vi "fileObjectivesRegistrationLoad.vi"(0 "objectiveRegistrationFilePath":string) -> (4 "denormParam":dbl[](array[numeric]), 5 "z(opto)z(img)":dbl[][](array[numeric]), 6 "param":dbl[](array[numeric]), 7 "imaging (model)":dbl[][](array[numeric]), 8 "normParam":dbl[](array[numeric]), 9 "optogenetics (scene)":dbl[][](array[numeric]))   [LabVIEW 2017]
uses:
  <vilib>/Utility/file.llb/Read Delimited Spreadsheet (DBL).vi
  <vilib>/Analysis/polynomials.llb/1D Polynomial Evaluation (DBL).vi
  globalUtilities.vi
  <vilib>/Analysis/NI_AALPro.lvlib
panel:
  out "Array":dbl[][][](array[numeric])
  out "f":string
  out "XY Graph":T1(graph)
  out "dtp1(dpt0)":dbl[](array[numeric])
  out "dtp0(dpt1)":dbl[](array[numeric])
  # "a1"
  # "a0"
  # "a2"
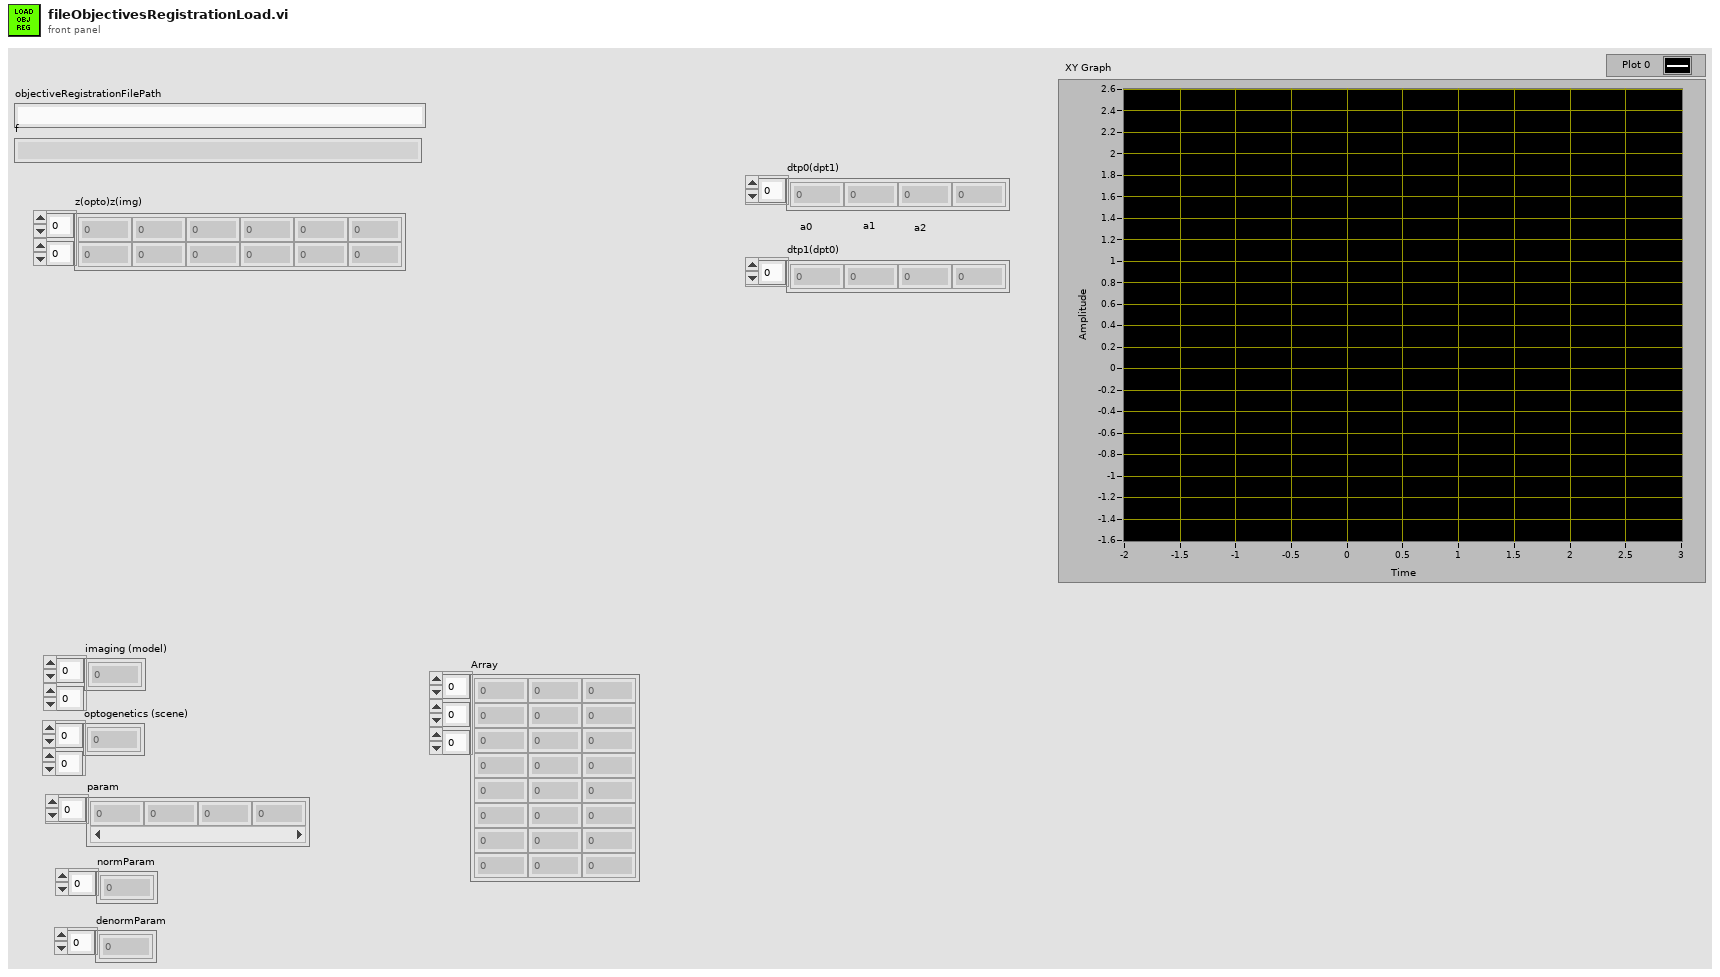
[diagram p1: front panel]
types:
  T1 = cluster{"all rows":dbl[], "Best Polynomial Fit":dbl[]}[]
  T2 = cluster{"all rows":dbl[], "Best Polynomial Fit":dbl[]}
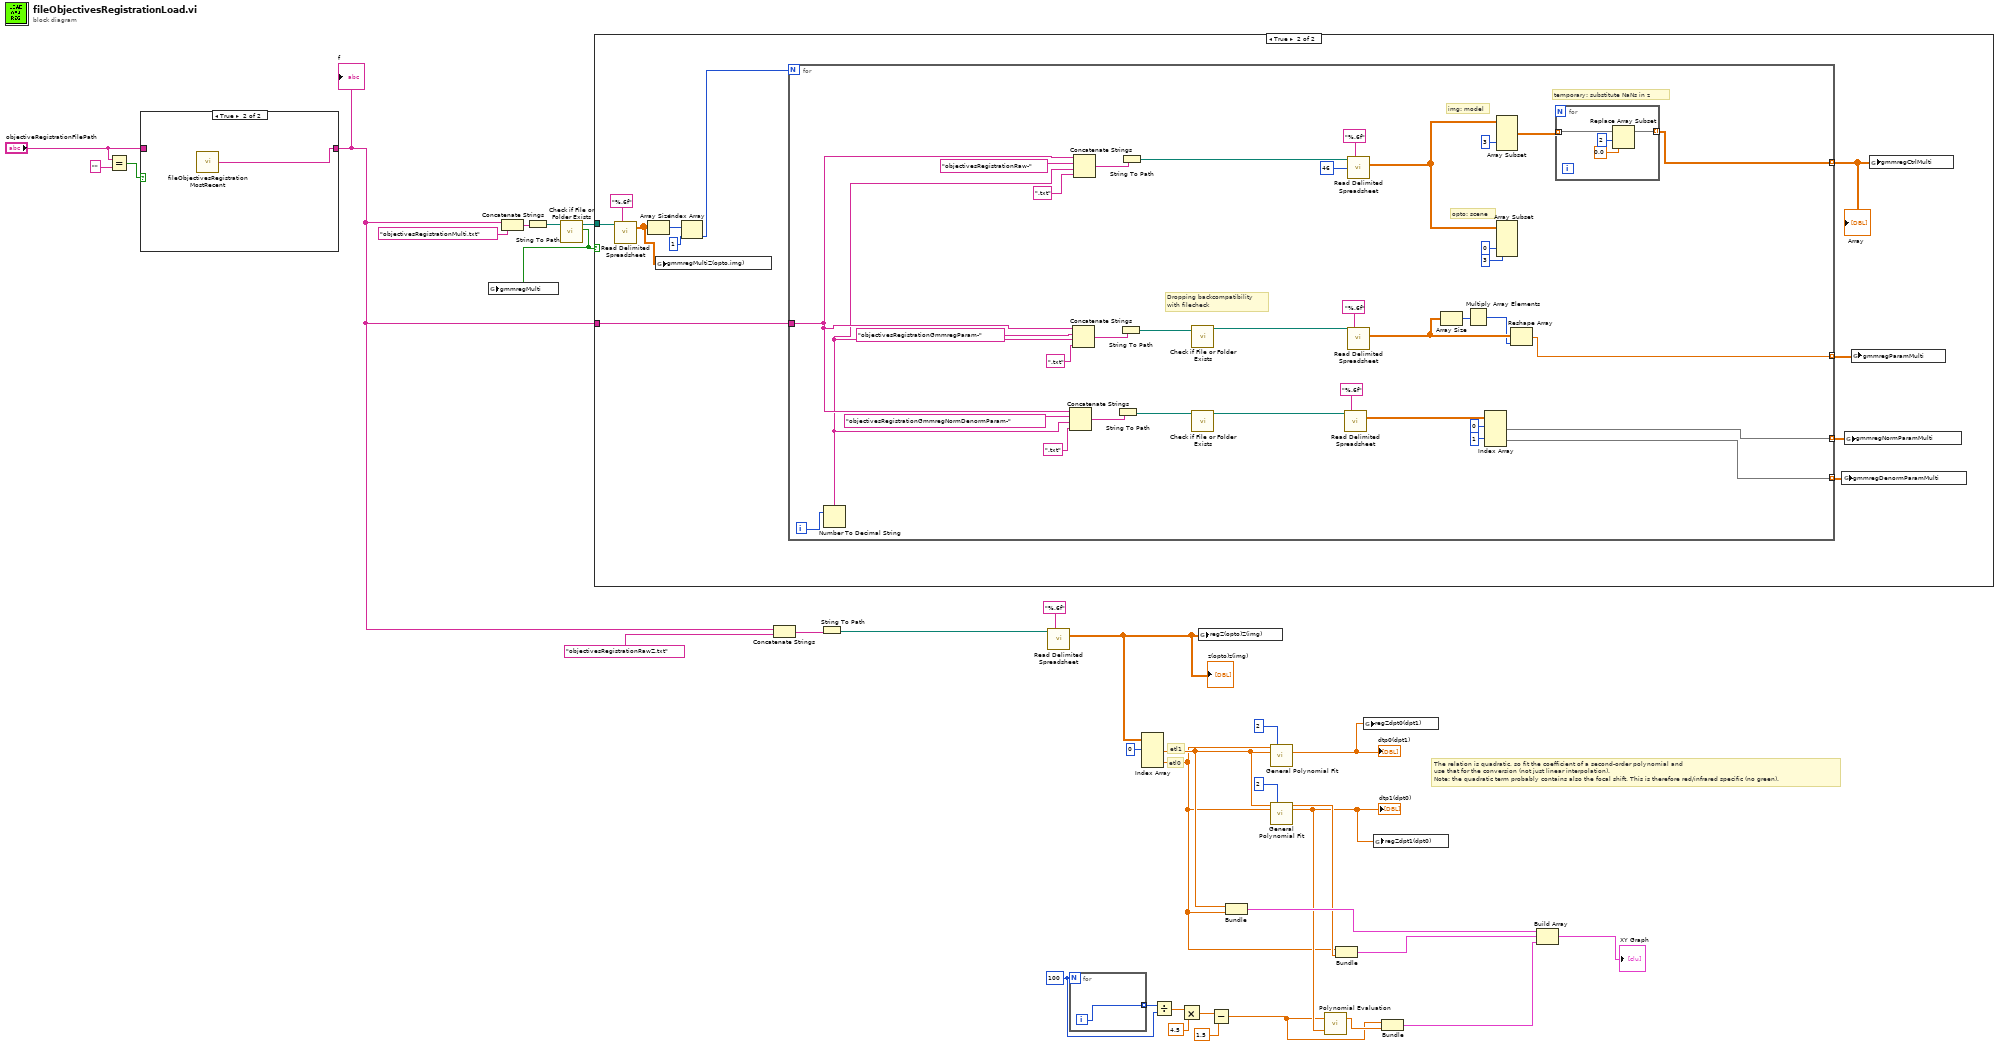
[diagram p0: block diagram]
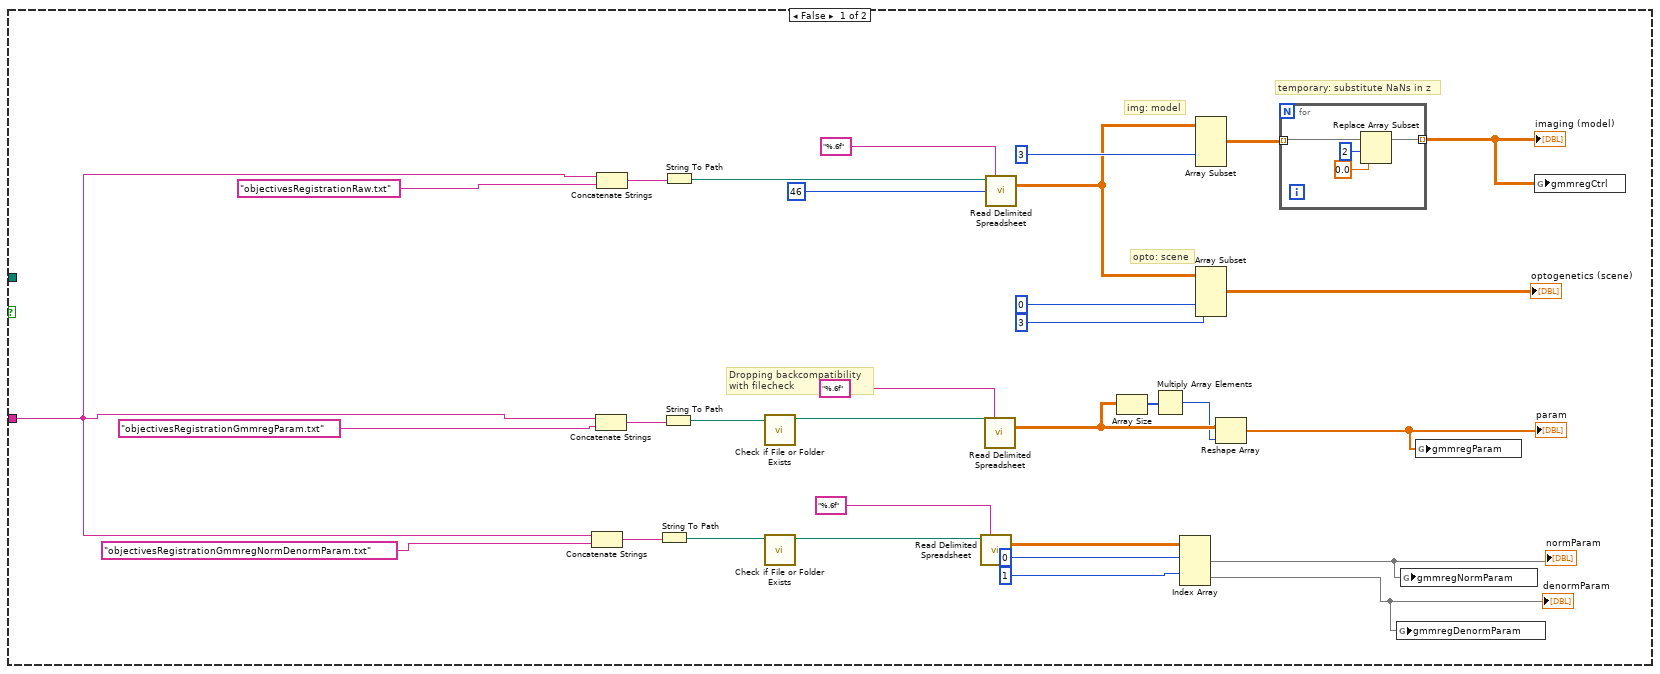
[diagram p2: hidden frame]
diagram:
  w19 = 100
  # "etl0"
  # "etl1"
  # "The relation is quadratic, so fit the coefficient of a second-order polynomial and\nuse that for the conversion (not just linear interpolation).\nNote: the quadratic term probably contains also the focal shift. This is therefore red/infrared specific (no green)."
  n1 = Equal?(x="objectiveRegistrationFilePath", y="") -> (x = y?=w11:bool)
  n2 = case shown="True" w11 {
    tunnel: "objectiveRegistrationFilePath" -> [w35 _]
    tunnel: [w35 w36] -> w4
    frame False {
    }
    frame True {
      n3 = call "fileObjectivesRegistrationMostRecent.vi"() -> ("f"=w36:string)  [unwired: 1 in]
    }
  }
  "f" <- w4
  n4 = Concatenate Strings(w4, "objectivesRegistrationMulti.txt") -> (w6:string)
  n5 = String To Path(string=w6) -> (path=w3:path)
  n6 = call <vilib>:"Check if File or Folder Exists.vi"("path"=w3) -> ("file or folder exists?"=w1:bool, "dup path"=w2:path)  [unwired: 8 in, 1 out]
  n7 = global write "globalUtilities.vi" "gmmregMulti"(w1) -> ()
  n8 = case shown="True" w1 {
    tunnel: w4 -> [w48 w83]
    tunnel: w2 -> [_ w81]
    frame False {
      # "Dropping backcompatibility\nwith filecheck"
      # "temporary: substitute NaNs in z"
      # "img: model"
      # "opto: scene"
      n9 = Concatenate Strings(w48, "objectivesRegistrationGmmregNormDenormParam.txt" ("string")) -> (w55:string)
      n10 = Concatenate Strings(w48, "objectivesRegistrationGmmregParam.txt" ("string")) -> (w57:string)
      n11 = Concatenate Strings(w48, "objectivesRegistrationRaw.txt" ("string")) -> (w58:string)
      n12 = String To Path(string=w55) -> (path=w52:path)
      n13 = String To Path(string=w57) -> (path=w53:path)
      n14 = String To Path(string=w58) -> (path=w60:path)
      n15 = call <vilib>:"Check if File or Folder Exists.vi"("path"=w53) -> ("dup path"=w51:path)  [unwired: 8 in, 2 out]
      n16 = call <vilib>:"Check if File or Folder Exists.vi"("path"=w52) -> ("dup path"=w50:path)  [unwired: 8 in, 2 out]
      n17 = call-poly <vilib>:"Read Delimited Spreadsheet.vi"("file path (dialog if empty)"=w50, "format (%.3f)"="%.6f") -> ("all rows"=w41:dbl[][])  [unwired: 8 in, 5 out]
      n18 = call-poly <vilib>:"Read Delimited Spreadsheet.vi"("file path (dialog if empty)"=w51, "format (%.3f)"="%.6f") -> ("all rows"=w45:dbl[][])  [unwired: 8 in, 5 out]
      n19 = call-poly <vilib>:"Read Delimited Spreadsheet.vi"("file path (dialog if empty)"=w60, "format (%.3f)"="%.6f", "start of read offset (chars.:0)"=46) -> ("all rows"=w63:dbl[][])  [unwired: 7 in, 5 out]
      n20 = Array Size(array=w45) -> (size(s)=w46:i32[])
      n21 = Multiply Array Elements(1:w46) -> (0:w44:i32)
      n22 = Index Array(array=w41, index (row) #1=0 ("index (row)"), index (row) #2=1 ("disabled index (col)")) -> (element #1=w38:dbl[], element #2=w37:dbl[])  [unwired: 2 in]
      "normParam" <- w38
      "denormParam" <- w37
      n23 = Array Subset(array=w63, index (col)=3 ("index")) -> (w62:dbl[][])  [unwired: 3 in]
      n24 = Array Subset(array=w63, index (col)=0 ("index"), length (col)=3 ("length")) -> (→"optogenetics (scene)":dbl[][])  [unwired: 2 in]
      n25 = Reshape Array(w45, w44) -> (w43:dbl[])
      "param" <- w43
      n26 = for {
        tunnel: w62 -> [w72] mode=indexing
        tunnel: [w69] -> w49 mode=indexing
        n27 = Replace Array Subset(array=w72, new element=0.0 ("new element/subarray"), index=2) -> (w69:dbl[])
      }
      "imaging (model)" <- w49
      n28 = global write "globalUtilities.vi" "gmmregDenormParam"(w37) -> ()
      n29 = global write "globalUtilities.vi" "gmmregNormParam"(w38) -> ()
      n30 = global write "globalUtilities.vi" "gmmregParam"(w43) -> ()
      n31 = global write "globalUtilities.vi" "gmmregCtrl"(w49) -> ()
    }
    frame True {
      n32 = call-poly <vilib>:"Read Delimited Spreadsheet.vi"("file path (dialog if empty)"=w81, "format (%.3f)"="%.6f") -> ("all rows"=w73:dbl[][])  [unwired: 8 in, 5 out]
      n33 = Array Size(array=w73) -> (size(s)=w80:i32[])
      n34 = global write "globalUtilities.vi" "gmmregMultiZ(opto,img)"(w73) -> ()
      n35 = Index Array(array=w80, index=1) -> (element=w78:i32)
      n36 = for {
        N: w78 -> [_]
        tunnel: w83 -> [w93]
        tunnel: [w87] -> w77 mode=indexing
        tunnel: [w86] -> w76 mode=indexing
        tunnel: [w85] -> w75 mode=indexing
        tunnel: [w84] -> w74 mode=indexing
        i -> [w89]
        # "Dropping backcompatibility\nwith filecheck"
        # "temporary: substitute NaNs in z"
        # "img: model"
        # "opto: scene"
        n37 = Number To Decimal String(number=w89) -> (decimal integer string=w88:string)  [unwired: 1 in]
        n38 = Concatenate Strings(w93, "objectivesRegistrationGmmregNormDenormParam-" ("string"), w88, ".txt" ("string")) -> (w107:string)
        n39 = Concatenate Strings(w93, "objectivesRegistrationGmmregParam-" ("string"), w88, ".txt" ("string")) -> (w109:string)
        n40 = Concatenate Strings(w93, "objectivesRegistrationRaw-" ("string"), w88, ".txt" ("string")) -> (w110:string)
        n41 = String To Path(string=w107) -> (path=w104:path)
        n42 = String To Path(string=w109) -> (path=w105:path)
        n43 = String To Path(string=w110) -> (path=w112:path)
        n44 = call <vilib>:"Check if File or Folder Exists.vi"("path"=w105) -> ("dup path"=w103:path)  [unwired: 8 in, 2 out]
        n45 = call <vilib>:"Check if File or Folder Exists.vi"("path"=w104) -> ("dup path"=w102:path)  [unwired: 8 in, 2 out]
        n46 = call-poly <vilib>:"Read Delimited Spreadsheet.vi"("file path (dialog if empty)"=w102, "format (%.3f)"="%.6f") -> ("all rows"=w96:dbl[][])  [unwired: 8 in, 5 out]
        n47 = call-poly <vilib>:"Read Delimited Spreadsheet.vi"("file path (dialog if empty)"=w103, "format (%.3f)"="%.6f") -> ("all rows"=w99:dbl[][])  [unwired: 8 in, 5 out]
        n48 = call-poly <vilib>:"Read Delimited Spreadsheet.vi"("file path (dialog if empty)"=w112, "format (%.3f)"="%.6f", "start of read offset (chars.:0)"=46) -> ("all rows"=w114:dbl[][])  [unwired: 7 in, 5 out]
        n49 = Array Size(array=w99) -> (size(s)=w100:i32[])
        n50 = Multiply Array Elements(1:w100) -> (0:w98:i32)
        n51 = Index Array(array=w96, index (row) #1=0 ("index (row)"), index (row) #2=1 ("disabled index (col)")) -> (element #1=w85:dbl[], element #2=w84:dbl[])  [unwired: 2 in]
        n52 = Array Subset(array=w114, index (col)=3 ("index")) -> (w113:dbl[][])  [unwired: 3 in]
        n53 = Array Subset(array=w114, index (col)=0 ("index"), length (col)=3 ("length")) -> ()  [unwired: 2 in, 1 out]
        n54 = Reshape Array(w99, w98) -> (w86:dbl[])
        n55 = for {
          tunnel: w113 -> [w123] mode=indexing
          tunnel: [w120] -> w87 mode=indexing
          n56 = Replace Array Subset(array=w123, new element=0.0 ("new element/subarray"), index=2) -> (w120:dbl[])
        }
      }
      "Array" <- w77
      n57 = global write "globalUtilities.vi" "gmmregDenormParamMulti"(w74) -> ()
      n58 = global write "globalUtilities.vi" "gmmregNormParamMulti"(w75) -> ()
      n59 = global write "globalUtilities.vi" "gmmregParamMulti"(w76) -> ()
      n60 = global write "globalUtilities.vi" "gmmregCtrlMulti"(w77) -> ()
    }
  }
  n61 = Concatenate Strings(w4, "objectivesRegistrationRawZ.txt" ("string")) -> (w34:string)
  n62 = String To Path(string=w34) -> (path=w32:path)
  n63 = call-poly <vilib>:"Read Delimited Spreadsheet.vi"("file path (dialog if empty)"=w32, "format (%.3f)"="%.6f") -> ("all rows"=w30:dbl[][])  [unwired: 8 in, 5 out]
  "z(opto)z(img)" <- w30
  n64 = for {
    N: w19 -> [_]
    tunnel: [w124] -> w20 mode=indexing
    i -> [w124]
  }
  n65 = Index Array(array=w30, index (row) #1=0 ("index (row)")) -> (element #1=w10:dbl[], element #2=w9:dbl[])  [unwired: 3 in]
  n66 = Divide(x=w20, y=w19) -> (x/y=w18:dbl[])
  n67 = Multiply(x=w18, y=4.5) -> (x*y=w16:dbl[])
  n68 = global write "globalUtilities.vi" "regZ(opto)Z(img)"(w30) -> ()
  n69 = Subtract(x=w16, y=1.5) -> (x-y=w14:dbl[])
  n70 = Bundle("all rows"=w10, "all rows"=w9) -> (w25:cluster{"all rows":dbl[], "all rows":dbl[]})  [unwired: 1 in]
  n71 = call <vilib>:"General Polynomial Fit.vi"("Y"=w9, "polynomial order"=2, "X"=w10) -> ("Polynomial Coefficients"=w26:dbl[])  [unwired: 9 in, 3 out]
  "dtp0(dpt1)" <- w26
  n72 = call <vilib>:"General Polynomial Fit.vi"("Y"=w10, "polynomial order"=2, "X"=w9) -> ("Best Polynomial Fit"=w23:dbl[], "Polynomial Coefficients"=w22:dbl[])  [unwired: 9 in, 2 out]
  "dtp1(dpt0)" <- w22
  n73 = call-poly <vilib>:"Polynomial Evaluation.vi"("P(x)"=w22, "A"=w14) -> ("P(A)"=w21:dbl[])  [unwired: 1 out]
  n74 = Bundle("all rows"=w9, "Best Polynomial Fit"=w23) -> (w8:T2)  [unwired: 1 in]
  n75 = global write "globalUtilities.vi" "regZdpt0(dpt1)"(w26) -> ()
  n76 = global write "globalUtilities.vi" "regZdpt1(dpt0)"(w22) -> ()
  n77 = Bundle(w14, "P(A)"=w21) -> (w7:cluster{dbl[], "P(A)":dbl[]})  [unwired: 1 in]
  n78 = Build Array(w25, w8, w7) -> (→"XY Graph":cluster{"all rows":dbl[], "P(A)":dbl[]}[])
